vi "MAIN_STANDALONE.vi"() -> ()   [LabVIEW 2019]
uses:
  VI's/ESTADOS_ABS.ctl
  <vilib>/Instr/_visa.llb/VISA Configure Serial Port (Instr).vi
  <vilib>/Utility/error.llb/Error Cluster From Error Code.vi
  <vilib>/ErrorRing/Error Ring.xnode
  SHARED VI'S/SHARED VI'S.lvlib
panel:
  in  "Tab depuracion":enum32{"Page 1", "Page 2"}(tab)
  in  "error in (no error)":errorcluster
  out "error out":errorcluster
  in  "Tab Control":enum32{"Page 2"}(tab)
  in  "START":bool
  in  "home":bool
  in  "stop":bool
  in  "PARÁMETROS ENTRADA":T1={"mm en X"=308.5, "mm en Y"=455.0, "mm en Z"=0.0} {"mm en Z" min=0.0 max=40.0; "mm en Y" min=100.0 max=550.0; "mm en X" min=90.0 max=650.0}
  out "ESTADO ACTUAL":T2
  # "EXISTEN LIMITES DE SEGURIDAD PARA LOS CONTROLES  en mm X,Y,Z \nNO MODIFICARLOS!!"
  # "/* Teoricamente en X e Y:\n1mm= 91,32 pasos\n1cm = 913,2 pasos\n10 cm = 9132 pasos\n0.1 mm = 9,132 pasos aprox\n*/\nEl eje Z se mueve 1 mm por cada 3200 pulsos.\nDesde la ventosa en posicion zero hasta el tablero metalico hay aprox. 45mm =144000 pulsos teoricamente.\nNO PONER NUNCA ÉSTE VALOR"
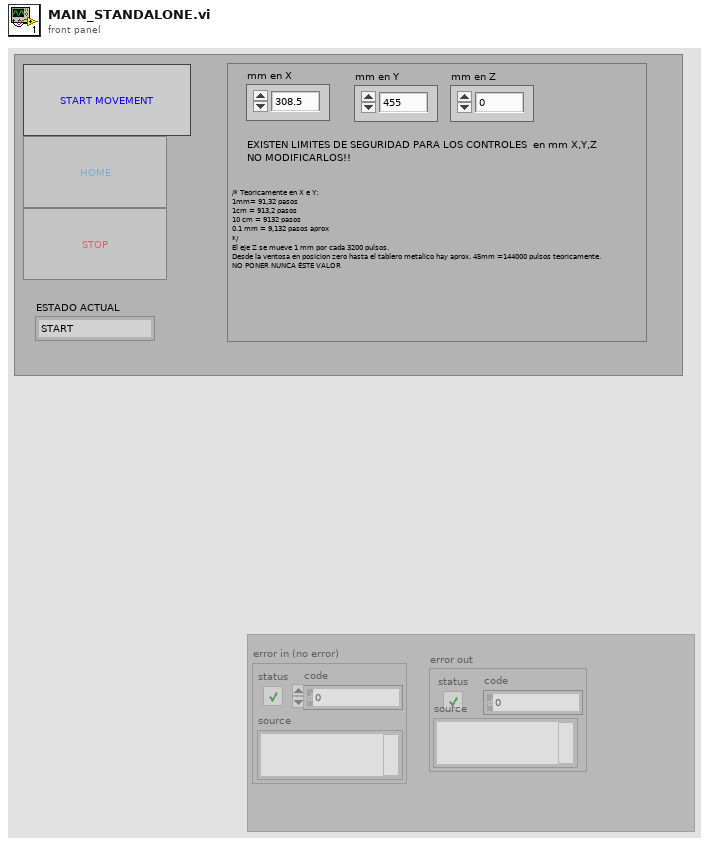
[diagram p1: front panel]
types:
  T1 = typedef "PARÁMETROS_ABSOLUTOS.ctl" = cluster{"mm en X":dbl, "mm en Y":dbl, "mm en Z":dbl}
  T2 = typedef "ESTADOS_ABS.ctl" = enum16{"START", "GESTION EVENTOS", "ENVIAR PARAMETROS", "HOME", "ERROR?", "SALIR"}
  T3 = enum8{"Enabled", "Disabled", "Disabled and Grayed Out"}
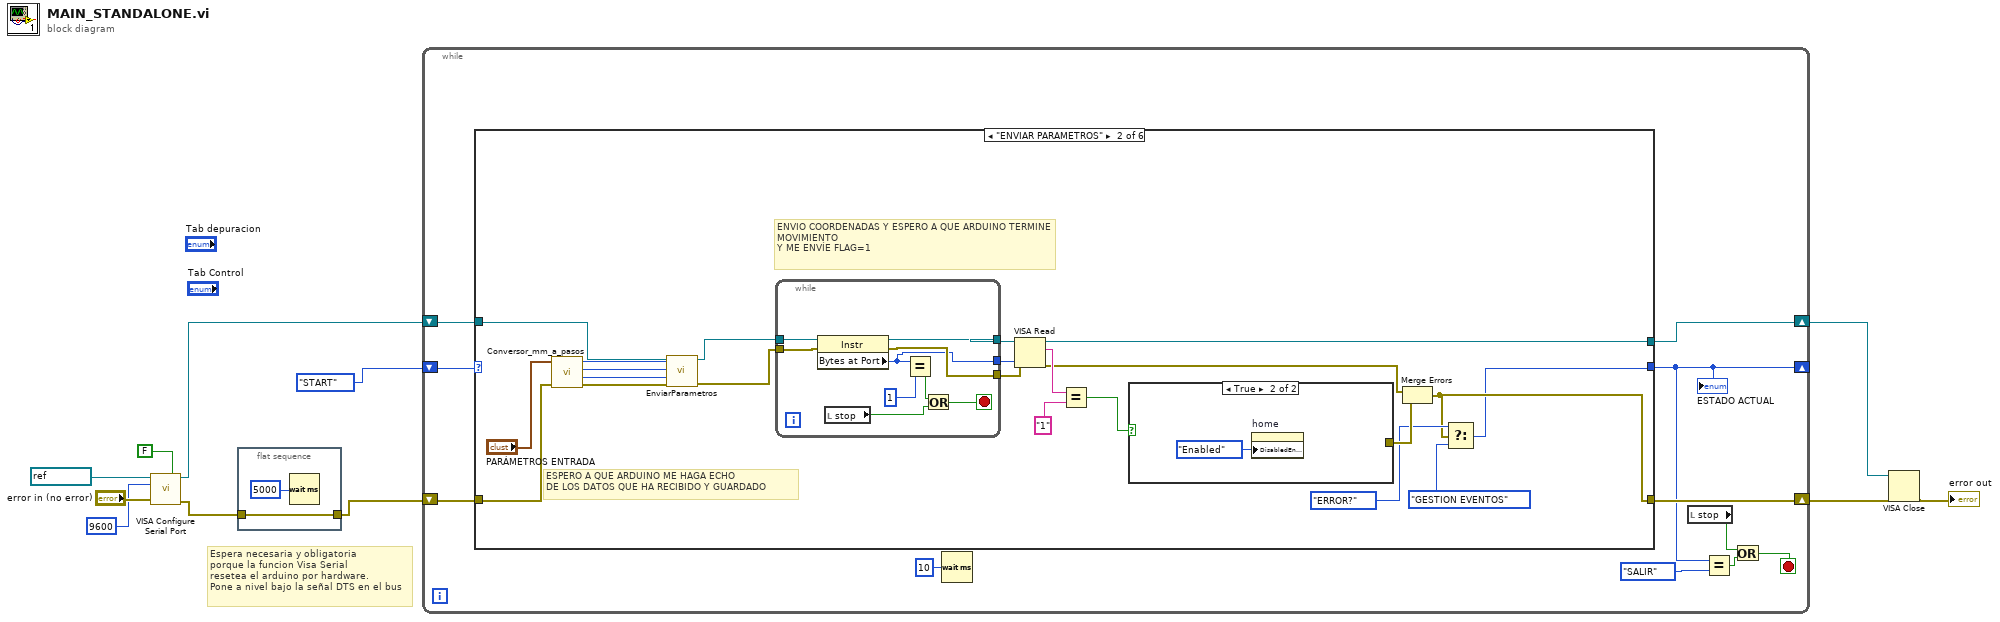
[diagram p0: block diagram]
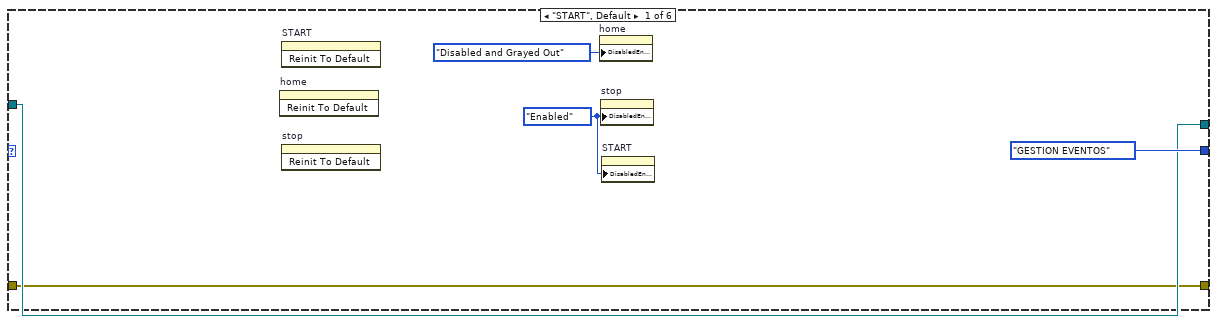
[diagram p2: hidden frame]
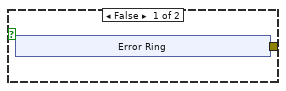
[diagram p3: hidden frame]
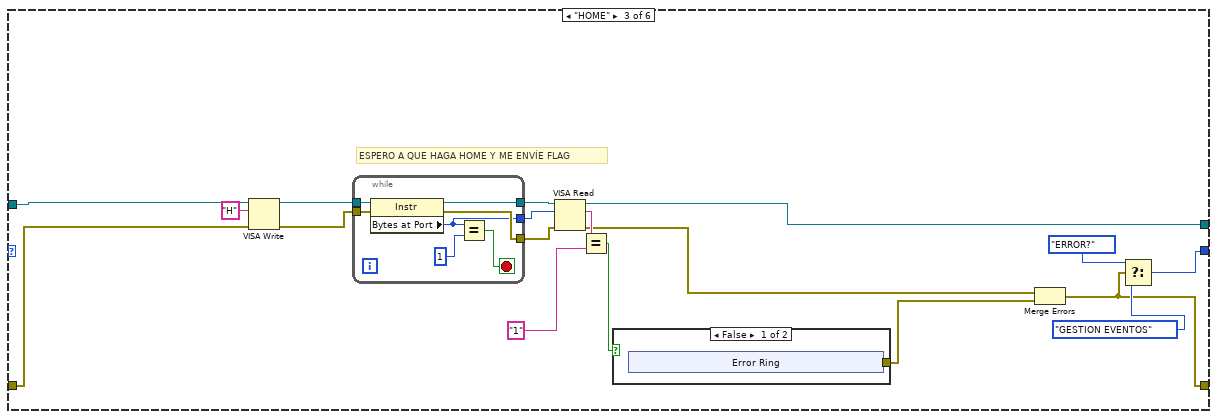
[diagram p4: hidden frame]
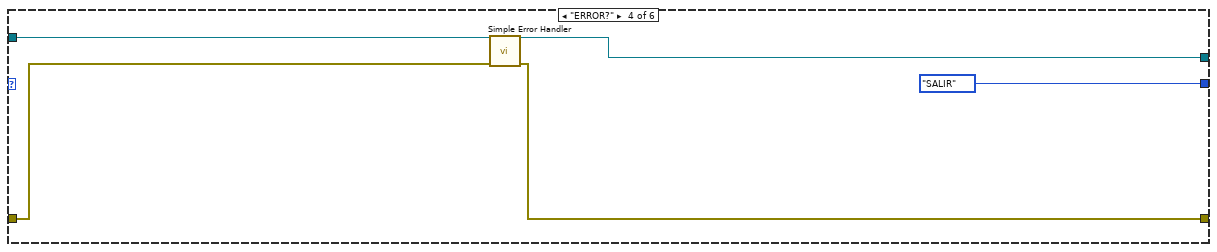
[diagram p6: hidden frame]
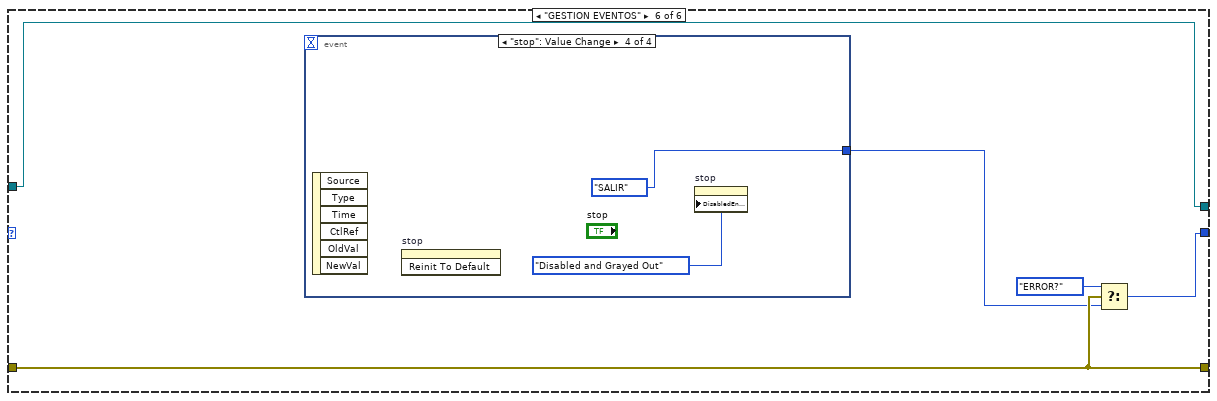
[diagram p8: hidden frame]
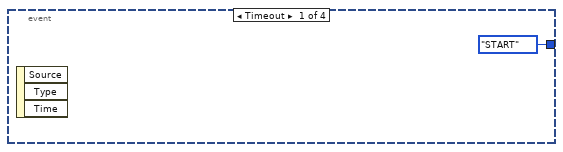
[diagram p9: hidden frame]
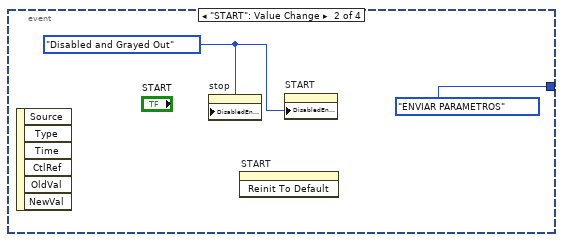
[diagram p10: hidden frame]
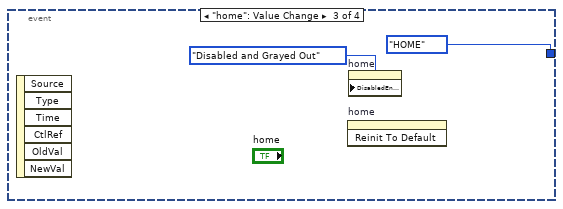
[diagram p11: hidden frame]
diagram:
  # "Espera necesaria y obligatoria\nporque la funcion Visa Serial\nresetea el arduino por hardware.\nPone a nivel bajo la señal DTS en el bus"
  n1 = call-poly "VISA Configure Serial Port"("VISA resource name"=refnum<visa-resource-name> "COM4", "Enable Termination\nChar (T)"=FALSE ("Enable Termination\nChar (T)"), "baud rate (9600)"=u32 9600, "error in (no error)"="error in (no error)") -> ("VISA resource name out"=w7:refnum<visa-resource-name>, "error out"=w4:errorcluster)  [unwired: 10 in]
  n2 = flat-sequence {
    tunnel: w4 -> [w12]
    tunnel: [w12] -> w3
    frame #0 {
      n3 = Wait (ms)(milliseconds to wait=u32 5000) -> ()  [unwired: 1 out]
    }
  }
  n4 = while {
    shift-right: [w17] -> _
    shift-left: ESTADOS_ABS."START" -> [w24]
    shift-right: [w19] -> w6
    shift-left: w3 -> [w23]
    shift-right: [w14] -> w1
    shift-left: w7 -> [w22]
    stop <- w20 stop-if-true
    n5 = case shown="\"ENVIAR PARAMETROS\"" w24 {
      selector: w24 -> [_ _ _ _ w104 _]
      tunnel: [ESTADOS_ABS."GESTION EVENTOS" ("t") w40 w72 ESTADOS_ABS."SALIR" w104 w108] -> w17
      tunnel: w23 -> [w27 w37 w84 w101 w103 w107]
      tunnel: w22 -> [w28 w32 w85 w102 w105 w110]
      tunnel: [w28 w47 w75 w102 w105 w110] -> w14
      tunnel: [w27 w41 w69 w100 w103 w107] -> w19
      frame "START", Default {
        w25 = T3."Enabled" ("Disabled")
        n6 = invoke on="home" class="Bool" method="Reinit To Default"() -> ()  [unwired: 3 in, 3 out]
        n7 = invoke on="START" class="Bool" method="Reinit To Default"() -> ()  [unwired: 3 in, 3 out]
        n8 = invoke on="stop" class="Bool (strict)" method="Reinit To Default"() -> ()  [unwired: 3 in, 3 out]
        n9 = property on="home" class="Bool"("DisabledEnum"=T3."Disabled and Grayed Out" ("Disabled")) -> ()  [unwired: 2 in, 2 out]
        n10 = property on="stop" class="Bool (strict)"("DisabledEnum"=w25) -> ()  [unwired: 2 in, 2 out]
        n11 = property on="START" class="Bool"("DisabledEnum"=w25) -> ()  [unwired: 2 in, 2 out]
      }
      frame "ENVIAR PARAMETROS" {
        # "ESPERO A QUE ARDUINO ME HAGA ECHO\nDE LOS DATOS QUE HA RECIBIDO Y GUARDADO"
        # "ENVIO COORDENADAS Y ESPERO A QUE ARDUINO TERMINE MOVIMIENTO\nY ME ENVÍE FLAG=1"
        n12 = call "Conversor_mm_a_pasos.vi"("error in (no error)"=w37, "PARÁMETROS ENTRADA"="PARÁMETROS ENTRADA") -> ("error out"=w33:errorcluster, "PASOS EN Z"=w34:i32, "PASOS EN Y"=w35:i32, "PASOS EN X"=w36:i32)  [unwired: 6 in]
        n13 = call "EnviarParametros.vi"("VISA resource name"=w32, "PASOS EN X"=w36, "PASOS EN Y"=w35, "PASOS EN Z"=w34, "error in (no error)"=w33) -> ("VISA resource name 2"=w31:refnum<visa-resource-name>, "error out"=w30:errorcluster)  [unwired: 9 in]
        n14 = while {
          tunnel: [w66] -> w50
          tunnel: [w65] -> w49
          tunnel: [w64] -> w39
          tunnel: w31 -> [w63]
          tunnel: w30 -> [w62]
          stop <- w60 stop-if-true
          n15 = property class="Instr"(reference=w63, error in=w62) -> (reference out=w66:refnum<visa-resource-name>, error out=w65:errorcluster, "Bytes at Port"=w64:u32)
          n16 = local read "stop"() -> (w59:bool)
          n17 = Equal?(x=w64, y=u32 1) -> (x = y?=w61:bool)
          n18 = Or(x=w61, y=w59) -> (x .or. y?=w60:bool)
        }
        n19 = VISA Read(VISA resource name=w50, byte count=w39, error in (no error)=w49) -> (VISA resource name out=w47:refnum<visa-resource-name>, read buffer=w48:string, error out=w45:errorcluster)  [unwired: 1 out]
        n20 = Equal?(x=w48, y="1") -> (x = y?=w46:bool)
        n21 = case shown="True" w46 {
          tunnel: [w52 _] -> w44
          frame False {
            n22 = xnode "Error Ring"() -> ("error out"=w52:errorcluster)
          }
          frame True {
            n23 = property on="home" class="Bool"("DisabledEnum"=T3."Enabled" ("Disabled")) -> ()  [unwired: 2 in, 2 out]
          }
        }
        n24 = Merge Errors(w45, w44) -> (w41:errorcluster)
        n25 = Select(t=ESTADOS_ABS."ERROR?", s=w41, f=ESTADOS_ABS."GESTION EVENTOS") -> (s? t:f=w40:T2)
      }
      frame "HOME" {
        # "ESPERO A QUE HAGA HOME Y ME ENVÍE FLAG"
        n26 = VISA Write(VISA resource name=w85, write buffer="H", error in (no error)=w84) -> (VISA resource name out=w76:refnum<visa-resource-name>, error out=w77:errorcluster)  [unwired: 1 out]
        n27 = while {
          tunnel: [w96] -> w82
          tunnel: [w95] -> w81
          tunnel: w77 -> [w94]
          tunnel: w76 -> [w93]
          tunnel: [w92] -> w70
          stop <- w98 stop-if-true
          n28 = property class="Instr"(reference=w93, error in=w94) -> (reference out=w96:refnum<visa-resource-name>, error out=w95:errorcluster, "Bytes at Port"=w92:u32)
          n29 = Equal?(x=w92, y=u32 1) -> (x = y?=w98:bool)
        }
        n30 = VISA Read(VISA resource name=w82, byte count=w70, error in (no error)=w81) -> (VISA resource name out=w75:refnum<visa-resource-name>, read buffer=w80:string, error out=w73:errorcluster)  [unwired: 1 out]
        n31 = Equal?(x=w80, y="1") -> (x = y?=w79:bool)
        n32 = case shown="False" w79 {
          tunnel: [w86 _] -> w74
          frame False {
            n33 = xnode "Error Ring"() -> ("error out"=w86:errorcluster)
          }
          frame True {
          }
        }
        n34 = Merge Errors(w73, w74) -> (w69:errorcluster)
        n35 = Select(t=ESTADOS_ABS."ERROR?", s=w69, f=ESTADOS_ABS."GESTION EVENTOS") -> (s? t:f=w72:T2)
      }
      frame "ERROR?" {
        n36 = call <vilib>:"Simple Error Handler.vi"("error in (no error)"=w101) -> ("error out"=w100:errorcluster)  [unwired: 4 in, 4 out]
      }
      frame "SALIR" {
      }
      frame "GESTION EVENTOS" {
        n37 = event shown="[3] \"stop\": Value Change" {
          selector: _ -> [_ _ _ _]
          dyn-events: _ -> [_ _ _ _]
          timeout: _ -> [_ _ _ _]
          tunnel: [ESTADOS_ABS."START" ("t") ESTADOS_ABS."ENVIAR PARAMETROS" ESTADOS_ABS."HOME" ("t") ESTADOS_ABS."SALIR" ("t")] -> w106
          event Timeout {
            n38 = event-data() -> ()  [unwired: 1 in, 3 out]
          }
          event "START": Value Change {
            w112 = T3."Disabled and Grayed Out" ("Disabled")
            n39 = event-data() -> ()  [unwired: 1 in, 6 out]
            n40 = property on="stop" class="Bool (strict)"("DisabledEnum"=w112) -> ()  [unwired: 2 in, 2 out]
            n41 = invoke on="START" class="Bool" method="Reinit To Default"() -> ()  [unwired: 3 in, 3 out]
            n42 = property on="START" class="Bool"("DisabledEnum"=w112) -> ()  [unwired: 2 in, 2 out]
          }
          event "home": Value Change {
            n43 = event-data() -> ()  [unwired: 1 in, 6 out]
            n44 = invoke on="home" class="Bool" method="Reinit To Default"() -> ()  [unwired: 3 in, 3 out]
            n45 = property on="home" class="Bool"("DisabledEnum"=T3."Disabled and Grayed Out" ("Disabled")) -> ()  [unwired: 2 in, 2 out]
          }
          event "stop": Value Change {
            n46 = event-data() -> ()  [unwired: 1 in, 6 out]
            n47 = invoke on="stop" class="Bool (strict)" method="Reinit To Default"() -> ()  [unwired: 3 in, 3 out]
            n48 = property on="stop" class="Bool (strict)"("DisabledEnum"=T3."Disabled and Grayed Out" ("Disabled")) -> ()  [unwired: 2 in, 2 out]
          }
        }
        n49 = Select(t=ESTADOS_ABS."ERROR?", s=w107, f=w106) -> (s? t:f=w108:T2)
      }
    }
    "ESTADO ACTUAL" <- w17
    n50 = Wait (ms)(milliseconds to wait=u32 10) -> ()  [unwired: 1 out]
    n51 = local read "stop"() -> (w15:bool)
    n52 = Equal?(x=w17, y=ESTADOS_ABS."SALIR") -> (x = y?=w18:bool)
    n53 = Or(x=w15, y=w18) -> (x .or. y?=w20:bool)
  }
  n54 = VISA Close(VISA resource name=w1, error in (no error)=w6) -> (error out=→"error out":errorcluster)
